vi "Configure Trigger.vi"(8 "error in (no error)":errorcluster, 11 "FGen PXI Base CFG in":refnum<class "FGen PXI Base CFG.lvclass">) -> (0 "error out":errorcluster, 3 "FGen PXI Base CFG out":refnum<class "FGen PXI Base CFG.lvclass">)   [LabVIEW 2023, in "FGen PXI Base CFG.lvlib" / "FGen PXI Base CFG.lvclass"]
uses:
  FGen PXI Base CFG.lvclass
  FGen PXI Base CFG.lvclass/FGen PXI Base CFG.ctl
  6833aab5-89e2-4c30-8132-47a66f565ddb.vi
  <instrlib>/niFgen/niFgen.llb/niFgen_ctl Exported Signal Identifiers (Ring).ctl
  <instrlib>/niFgen/niFgen.llb/niFgen_ctl Exported Signal Name Values (Ring).ctl
  <instrlib>/niFgen/niFgen.llb/niFgen_ctl Exported Signal Desination Values (ComboBox).ctl
  <vilib>/ErrorRing/Error Ring.xnode
  <vilib>/Utility/error.llb/Error Cluster From Error Code.vi
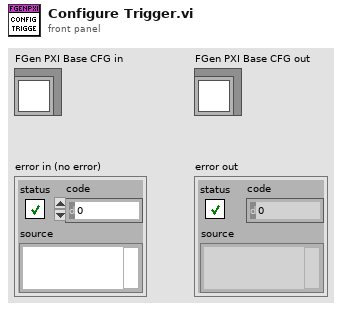
[diagram p1: front panel]
types:
  T1 = typedef "niFgen_ctl Exported Signal Desination Values (ComboBox).ctl" = string
  T2 = typedef "niFgen_ctl Exported Signal Identifiers (Ring).ctl" = string
  T3 = typedef "niFgen_ctl Exported Signal Name Values (Ring).ctl" = u16
  T4 = cluster{"Enabled":bool, "Output Terminal":T1, "Signal Identifier":T2, "Signal":T3}
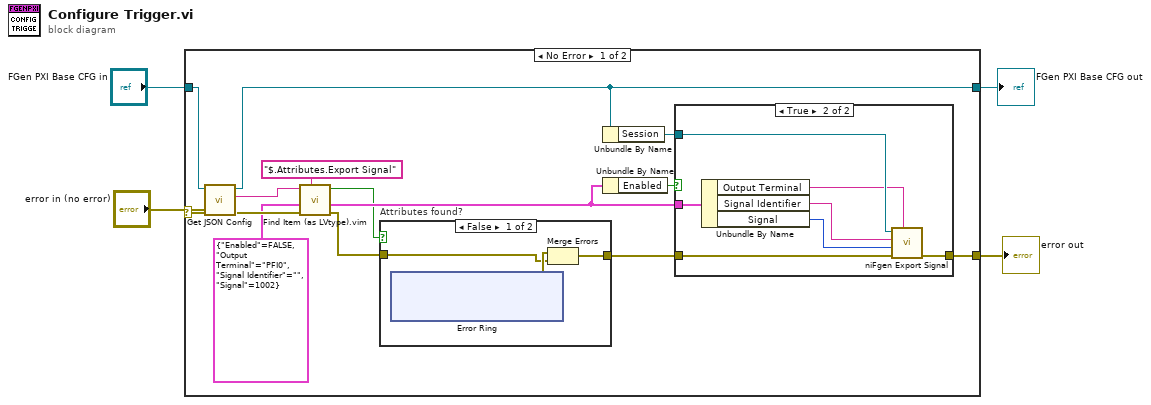
[diagram p0: block diagram]
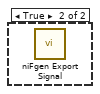
[diagram p2: hidden frame]
diagram:
  n1 = case shown="No Error" "error in (no error)" {
    selector: "error in (no error)" -> [w16 w40]
    tunnel: [w17 w40] -> w4
    tunnel: [w12 w39] -> w2
    tunnel: "FGen PXI Base CFG in" -> [w13 w39]
    frame No Error {
      n2 = call-dynamic "Get JSON Config.vi"("error in (no error)"=w16, "CFG Base in"=w13) -> ("error out"=w14:errorcluster, "<JSON>Config>"=w10:string, "CFG Base out"=w12:refnum<class "FGen PXI Base CFG.lvclass">)  [unwired: 7 in]
      n3 = call "Find Item (as LVtype).vim"("$Path or Item Name"="$.Attributes.Export Signal", "error in (no error)"=w14, "Data Type and Default Value"=T4 {"Enabled"=FALSE, "Output Terminal"="PFI0", "Signal Identifier"="", "Signal"=1002}, "JSON"=w10) -> ("error out"=w7:errorcluster, "Data"=w8:T4, "Found"=w6:bool)  [unwired: 4 in, 1 out]
      n4 = case "Attributes found?" shown="False" w6 {
        tunnel: [w20 _] -> w5
        tunnel: w7 -> [w19 _]
        frame False {
          n5 = xnode "Error Ring"() -> ("error out"=w21:errorcluster)
          n6 = Merge Errors(w21, w19) -> (w20:errorcluster)
        }
        frame True {
          n7 = call <instrlib>:"niFgen Export Signal.vi"() -> ("Output Terminal (do not export)"=w29:T1, "Signal"=w27:T3, "Signal Identifier (None)"=w28:T2, "Instrument Handle"=w30:refnum<k15>)  [unwired: 6 in, 2 out]
        }
      }
      n8 = Unbundle By Name(w12) -> ("Session"=w15:refnum<k15>)
      n9 = Unbundle By Name(w8) -> ("Enabled"=w9:bool)
      n10 = case shown="True" w9 {
        tunnel: [w31 w32] -> w17
        tunnel: w5 -> [w31 w37]
        tunnel: w8 -> [_ w38]
        tunnel: w15 -> [_ w34]
        frame False {
        }
        frame True {
          n11 = Unbundle By Name(w38) -> ("Output Terminal"=w33:T1, "Signal Identifier"=w35:T2, "Signal"=w36:T3)
          n12 = call <instrlib>:"niFgen Export Signal.vi"("Output Terminal (do not export)"=w33, "error in (no error)"=w37, "Signal"=w36, "Signal Identifier (None)"=w35, "Instrument Handle"=w34) -> ("error out"=w32:errorcluster)  [unwired: 5 in, 1 out]
        }
      }
    }
    frame Error {
    }
  }
  "error out" <- w4
  "FGen PXI Base CFG out" <- w2
